vi "FWHMCalculate.vi"(0 "Lambda":dbl[](array[numeric]), 1 "Spectra":dbl[](array[numeric])) -> (2 "Spectral Results":T1, 3 "Right Band":cluster{dbl[], dbl[]}, 4 "Left Band":cluster{dbl[], dbl[]})   [LabVIEW 2012]
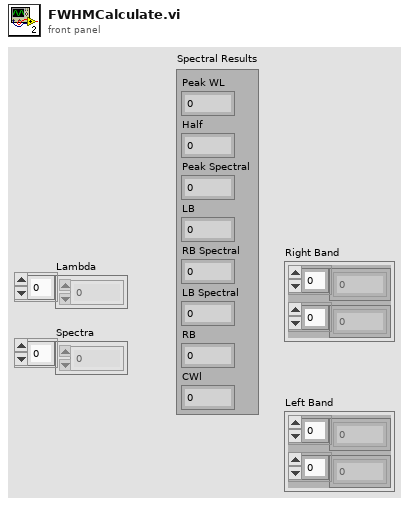
[diagram p1: front panel]
types:
  T1 = cluster{"Peak WL":dbl, "Half":dbl, "Peak Spectral":dbl, "LB":dbl, "RB Spectral":dbl, "LB Spectral":dbl, "RB":dbl, "CWl":dbl}
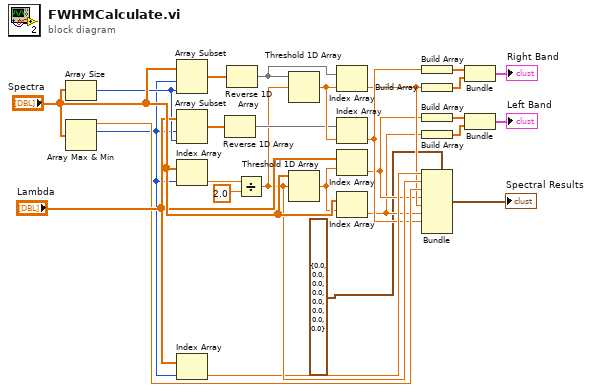
[diagram p0: block diagram]
diagram:
  n1 = Array Size(array="Spectra") -> (size(s)=w19:i32)
  n2 = Array Max & Min(array="Spectra") -> (max value=w9:dbl, max index (indices)=w8:i32)  [unwired: 2 out]
  n3 = Array Subset(array="Spectra", index=w8, length=w19) -> (w20:dbl[])
  n4 = Array Subset(array="Lambda", index=w8, length=w19) -> (w21:dbl[])
  n5 = Index Array(array="Spectra", index=w8) -> (element=w18:dbl)
  n6 = Index Array "Index Array"(array="Lambda", index=w8) -> (element=w7:dbl)
  n7 = Reverse 1D Array(array=w21) -> (reversed array=w22:dbl[])
  n8 = Reverse 1D Array(array=w20) -> (reversed array=w24:dbl[])
  n9 = Divide(x=w18, y=2.0) -> (x/y=w10:dbl)
  n10 = Threshold 1D Array(2:w10, 3:w24) -> (0:w23:dbl)  [unwired: 1 in]
  n11 = Threshold 1D Array(2:w10, 3:"Spectra") -> (0:w25:dbl)  [unwired: 1 in]
  n12 = Index Array(array=w24, index=w23) -> (element=w5:dbl)
  n13 = Index Array(array=w22, index=w23) -> (element=w6:dbl)
  n14 = Index Array(array="Lambda", index=w25) -> (element=w4:dbl)
  n15 = Index Array(array="Spectra", index=w25) -> (element=w3:dbl)
  n16 = Build Array(w6) -> (w16:dbl[])
  n17 = Build Array(w5) -> (w15:dbl[])
  n18 = Build Array(w4) -> (w13:dbl[])
  n19 = Build Array(w3) -> (w12:dbl[])
  n20 = Bundle(cluster=T1 {"Peak WL"=0.0, "Half"=0.0, "Peak Spectral"=0.0, "LB"=0.0, "RB Spectral"=0.0, "LB Spectral"=0.0, "RB"=0.0, "CWl"=0.0} ("Spectral Results"), "Peak WL"=w7, "Half"=w10, "Peak Spectral"=w9, "LB"=w4, "RB Spectral"=w5, "LB Spectral"=w3, "RB"=w6) -> (→"Spectral Results":T1)  [unwired: 1 in]
  n21 = Bundle(w16, w15) -> (→"Right Band":cluster{dbl[], dbl[]})  [unwired: 1 in]
  n22 = Bundle(w13, w12) -> (→"Left Band":cluster{dbl[], dbl[]})  [unwired: 1 in]
